vi "RichToFlatGreeter_req.vi"(5 "OutputClusterType":T1, 11 "InputCluster":T3) -> (3 "OutputCluster":T1)   [LabVIEW 2019, in "Generated_server.lvlib"]
uses:
  Generated_server.lvlib
  Greeter_req.ctl
  Greeter_req_req_oneof/Greeter_req_req_oneof.lvclass
  Greeter_req_Flat.ctl
  Greeter_MessageA_Flat.ctl
  Greeter_req_req_oneof/Greeter_req_req_oneof.lvclass/Greeter_req_req_oneof.ctl
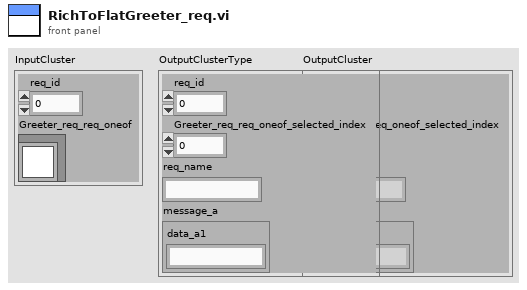
[diagram p1: front panel]
types:
  T1 = typedef "Generated_server.lvlib/Greeter_req_Flat.ctl" = cluster{"req_id":i32, "Greeter_req_req_oneof_selected_index":i32, "req_name":string, "message_a":T2}
  T2 = typedef "Generated_server.lvlib/Greeter_MessageA_Flat.ctl" = cluster{"data_a1":string}
  T3 = typedef "Generated_server.lvlib/Greeter_req.ctl" = cluster{"req_id":i32, "Greeter_req_req_oneof":refnum<class "Greeter_req_req_oneof.lvclass">}
  T4 = typedef "Generated_server.lvlib/Greeter_MessageA.ctl" = cluster{"data_a1":string}
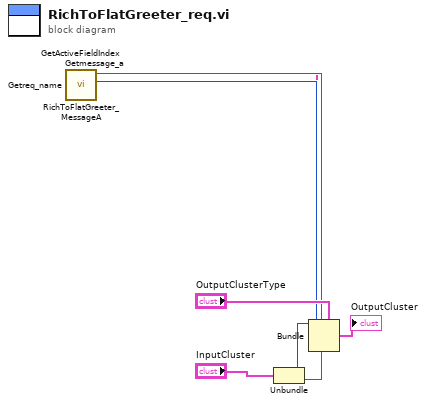
[diagram p0: block diagram]
diagram:
  n1 = Unbundle "Unbundle"("InputCluster") -> ("req_id"=w6:i32, "Greeter_req_req_oneof"=w5:refnum<class "Greeter_req_req_oneof.lvclass">)
  n2 = call "Getmessage_a.vi"("OneOfTemplate in"=w5) -> ("Get_Val"=w2:T4)  [unwired: 8 in, 2 out]
  n3 = call "RichToFlatGreeter_MessageA.vi"("InputCluster"=w2) -> ("OutputCluster"=w1:T2)  [unwired: 10 in]
  n4 = call "Getreq_name.vi"("OneOfTemplate in"=w5) -> ("Get_Val"=w3:string)  [unwired: 8 in, 2 out]
  n5 = call "GetActiveFieldIndex.vi"("OneOfTemplate in"=w5) -> ("Active Field Index"=w4:i32)  [unwired: 8 in, 2 out]
  n6 = Bundle "Bundle"(cluster="OutputClusterType", "req_id"=w6, "Greeter_req_req_oneof_selected_index"=w4, "req_name"=w3, "message_a"=w1) -> (→"OutputCluster":T1)
